vi "getLHeLevel.vi"(8 "error in (no error)":errorcluster, 11 "instrument.PPMS":refnum<class "instrument.PPMS.lvclass">) -> (0 "error out":errorcluster, 2 "LHe Level (%)":dbl, 3 "instrument.PPMS out":refnum<class "instrument.PPMS.lvclass">)   [LabVIEW 2019, in "instrument.PPMS.lvclass"]
uses:
  instrument.PPMS.lvclass
  <userlib>/LevyLab/Instrument Framework/Instrument Types/Cryostat/Instrument.Cryostat.lvclass
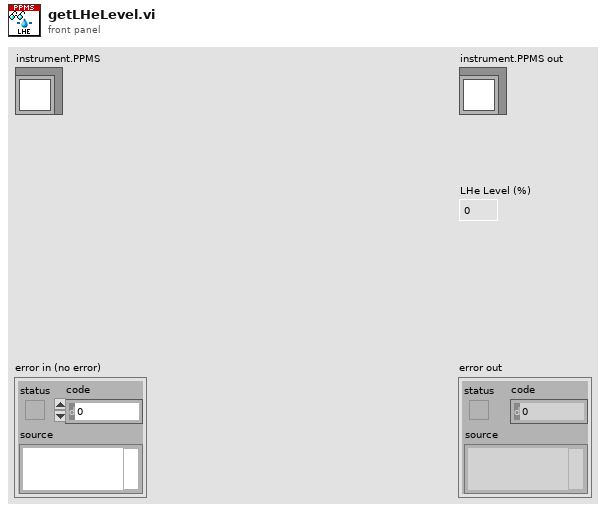
[diagram p1: front panel]
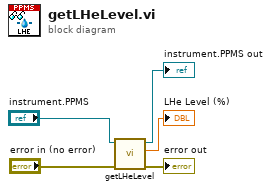
[diagram p0: block diagram]
diagram:
  n1 = call-parent "getLHeLevel.vi"("error in (no error)"="error in (no error)", "Instrument.Cryostat in"="instrument.PPMS") -> ("error out"=→"error out":errorcluster, "LHe Level (%)"=→"LHe Level (%)":dbl, "Instrument.Cryostat out"=→"instrument.PPMS out":refnum<class "instrument.PPMS.lvclass">)  [unwired: 7 in]
